vi "Read configuration.vi"(8 "error in (no error)":errorcluster, 11 "PS Channel":refnum<class "Power Supply Channel.lvclass">) -> (0 "error out":errorcluster, 2 "configuration":refnum<class "CEF_serializable configuration.lvclass">, 3 "PS Channel out":refnum<class "Power Supply Channel.lvclass">)   [LabVIEW 2025, in "Power Supply.lvlib" / "Power Supply Channel.lvclass"]
uses:
  Power Supply Channel.lvclass
  Users/Public/Documents/Sandia National Labs/TSS Plugin/CEF.lvlibp/serializable configuration/CEF_serializable configuration.lvclass
  Power Supply Channel.lvclass/Power Supply Channel.ctl
  PS Channel configuration/Power Supply Channel configuration.lvclass
  C:/Users/Public/Documents/Sandia National Labs/TSS Plugin/CEF.lvlibp/serializable configuration/CEF_serializable configuration.lvclass
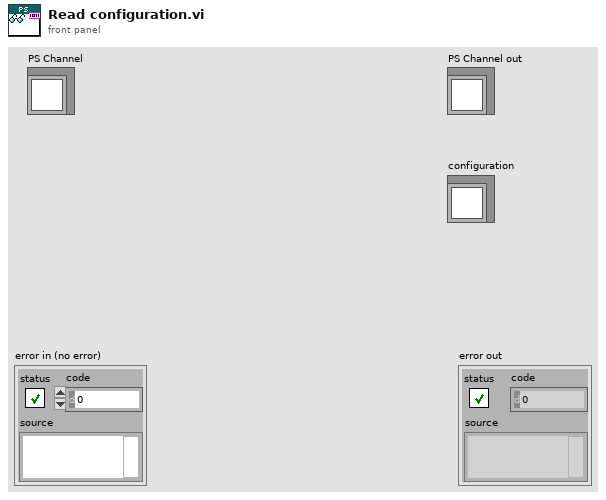
[diagram p1: front panel]
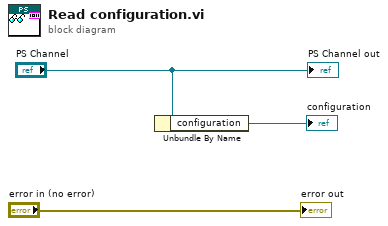
[diagram p0: block diagram]
diagram:
  n1 = Unbundle By Name("PS Channel") -> ("configuration"=→"configuration":refnum<class "Power Supply Channel configuration.lvclass">)
  "error out" <- "error in (no error)"
  "PS Channel out" <- "PS Channel"
